vi "load_enableChiller.vi"(8 "error in (no error)":errorcluster, 10 "start":bool, 11 "Instrument in":refnum<class "Instrument.lvclass">) -> (0 "error out":errorcluster, 3 "Instrument out":refnum<class "Instrument.lvclass">)   [LabVIEW 2019, in "Instrument.lvclass"]
uses:
  Instrument.lvclass
  Instrument.lvclass/Instrument.ctl
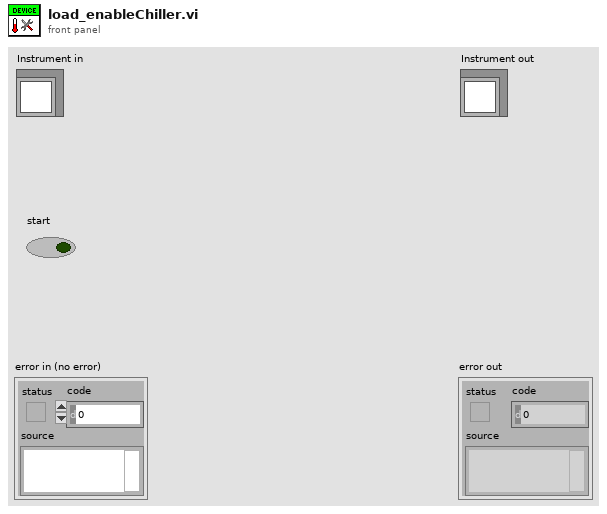
[diagram p1: front panel]
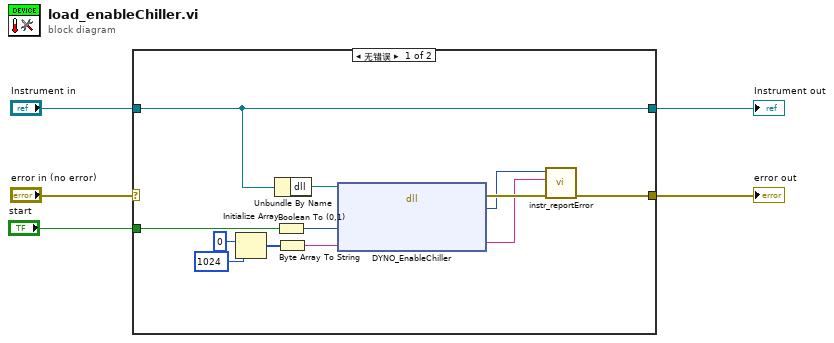
[diagram p0: block diagram]
diagram:
  n1 = case shown="无错误" "error in (no error)" {
    selector: "error in (no error)" -> [_ w19]
    tunnel: [w12 w19] -> w4
    tunnel: [w17 w18] -> w2
    tunnel: "Instrument in" -> [w17 w18]
    tunnel: "start" -> [w11 _]
    frame No Error {
      n2 = Initialize Array(u8 0 ("element"), 1024 ("dimension size")) -> (w7:u8[])
      n3 = Unbundle By Name(w17) -> ("dll"=w16:path)
      n4 = Boolean To (0,1)(Boolean=w11) -> (0, 1=w10:i16)
      n5 = Byte Array To String(unsigned byte array=w7) -> (string=w6:string)
      n6 = dll-call lib="C:/Dev/22KW-Dyno/software/data/DynoAPI.dll" fn="DYNO_EnableChiller"(path in=w16, "start"=w10, "errorMsg"=w6) -> (error out=w15:errorcluster, "return type"=w14:i32, "errorMsg"=w13:string)  [unwired: 3 in, 1 out]
      n7 = call "instr_reportError.vi"("error in (no error)"=w15, "errorMsg"=w13, "return type"=w14) -> ("error out"=w12:errorcluster)  [unwired: 8 in]
    }
    frame Error {
    }
  }
  "error out" <- w4
  "Instrument out" <- w2
